vi "set uart settings.vi"(8 "error in (no error)":errorcluster, 10 "uart_settings":cluster{"Speed":u32, "UARTSetupFlags":u32}, 11 "id":i32) -> (0 "error out":errorcluster, 3 "function return":i32)   [LabVIEW 2012, in "libximc.lvlib"]
doc: "result_t XIMC_API set_uart_settings (device_t id, const uart_settings_t* uart_settings);"
uses:
  libximc.lvlib
  libximc.dll
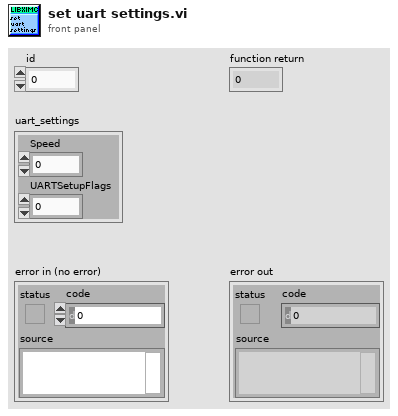
[diagram p1: front panel]
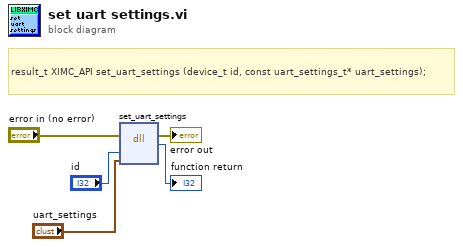
[diagram p0: block diagram]
diagram:
  # "result_t XIMC_API set_uart_settings (device_t id, const uart_settings_t* uart_settings);"
  n1 = dll-call lib="C:/Users/Stepan/Downloads/labview_2.9.11_testgen_thread/libximc.*" fn="set_uart_settings"(error in="error in (no error)", "id"="id", "uart_settings"="uart_settings") -> (error out=→"error out":errorcluster, →"function return":i32)  [unwired: 4 in, 1 out]
